vi "Magnitude.vi"(11 "Data in":dbl[][](array[numeric])) -> (1 "Phase":dbl[][](array[numeric]), 3 "Magnitude":dbl[][](array[numeric]), 4 "complex":cdb[][](array[numeric]))   [LabVIEW 2022 SP3]
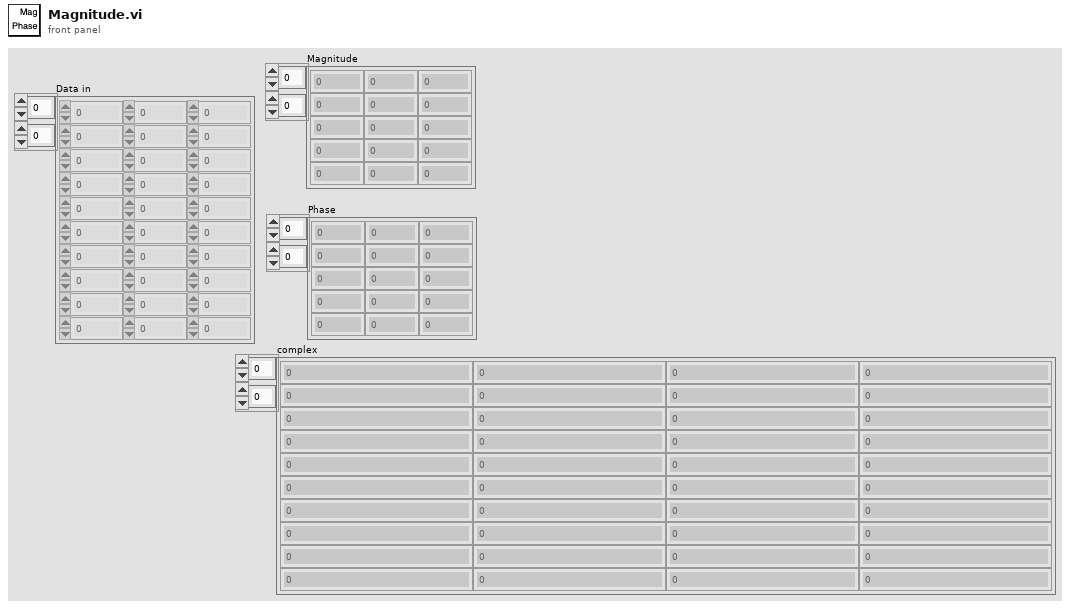
[diagram p1: front panel]
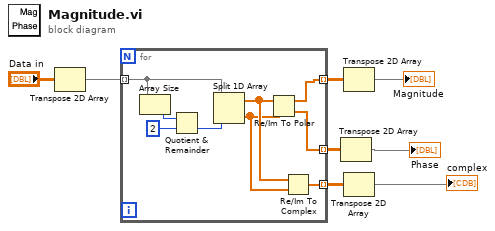
[diagram p0: block diagram]
diagram:
  n1 = Transpose 2D Array(2D array="Data in") -> (transposed array=w7:dbl[][])
  n2 = for {
    tunnel: w7 -> [w15] mode=indexing
    tunnel: [w17] -> w4 mode=indexing
    tunnel: [w16] -> w3 mode=indexing
    tunnel: [w9] -> w2 mode=indexing
    n3 = Array Size(array=w15) -> (size(s)=w14:i32)
    n4 = Quotient & Remainder(x=w14, y=2) -> (floor(x/y)=w12:i32)  [unwired: 1 out]
    n5 = Split 1D Array(array=w15, index=w12) -> (first subarray=w11:dbl[], second subarray=w10:dbl[])
    n6 = Re/Im To Polar(2:w10, 3:w11) -> (0:w16:dbl[], 1:w17:dbl[])
    n7 = Re/Im To Complex(1:w10, 2:w11) -> (0:w9:cdb[])
  }
  n8 = Transpose 2D Array(2D array=w3) -> (transposed array=→"Phase":dbl[][])
  n9 = Transpose 2D Array(2D array=w4) -> (transposed array=→"Magnitude":dbl[][])
  n10 = Transpose 2D Array(2D array=w2) -> (transposed array=→"complex":cdb[][])
